vi "Set VI Icon Demo.vi"() -> ()   [LabVIEW 2013]
panel:
  out "文件名":string[](array[string])
  in  "停止":bool
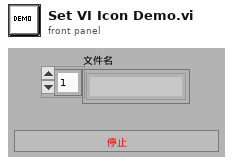
[diagram p1: front panel]
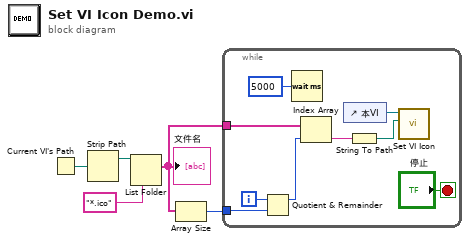
[diagram p0: block diagram]
diagram:
  n1 = Current VI's Path() -> (path=w2:path)
  n2 = Strip Path(path=w2) -> (stripped path=w3:path)  [unwired: 1 out]
  n3 = List Folder(path=w3, pattern="*.ico" ("模式")) -> (filenames=w4:string[])  [unwired: 2 in, 3 out]
  "文件名" <- w4
  n4 = Array Size(array=w4) -> (size(s)=w5:i32)
  n5 = while {
    tunnel: w5 -> [w11]
    tunnel: w4 -> [w10]
    i -> [w12]
    stop <- "停止" stop-if-true
    n6 = Quotient & Remainder(x=w12, y=w11) -> (x-y*floor(x/y)=w9:i32)  [unwired: 1 out]
    n7 = Wait (ms)(milliseconds to wait=u32 5000 ("毫秒倍数")) -> ()  [unwired: 1 out]
    n8 = Index Array(array=w10, index=w9) -> (element=w8:string)
    n9 = control-ref of="本VI"() -> (w6:refnum<vi>)
    n10 = String To Path(string=w8) -> (path=w7:path)
    n11 = call "Set VI Icon.vi"("路径"=w7, "VI引用句柄"=w6) -> ()  [unwired: 8 in, 2 out]
  }
